vi "read2Bytes.vi"(2 "Indice in":i32, 3 "Byte array":u8[](array[numeric])) -> (0 "Output":u16, 1 "Indice out":i32)   [LabVIEW 2014]
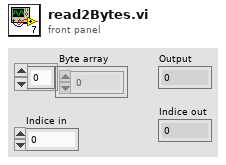
[diagram p1: front panel]
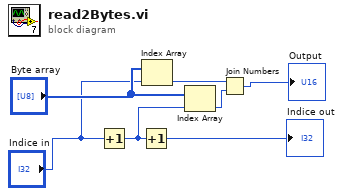
[diagram p0: block diagram]
diagram:
  n1 = Increment(x="Indice in") -> (x+1=w2:i32)
  n2 = Increment(x=w2) -> (x+1=→"Indice out":i32)
  n3 = Index Array(array="Byte array", index="Indice in") -> (element=w5:u8)
  n4 = Index Array(array="Byte array", index=w2) -> (element=w4:u8)
  n5 = Join Numbers(hi=w5, lo=w4) -> ((hi.lo)=→"Output":u16)
